vi "Octave Band Frequencies List.vi"(4 "high band selector":i32, 5 "low band selector":i32, 6 "bandwidth":T3(ring)=enum."1/3 octave", 7 "standard":T1) -> (0 "number of bands":i32, 1 "bandedge frequencies [Hz]":T2(array[cluster]) {"midband" format="%.2f"; "f high" format="%.2f"; "f low" format="%.2f"}, 2 "nominal frequencies (string)":string[](array[string]), 3 "nominal frequencies [Hz]":dbl[](array[numeric]) format="%.2f")   [LabVIEW 2017]
doc: "Returns nominal, or preferred, frequencies and bandedge frequencies based on the specified standard (ANSI or IEC), bandwidth, and low and high band selectors.\nThe frequency range is based on the low and high band selectors. A value of 0 corresponds to the reference frequency of the audio-frequency range, 1 kHz. Each successive value corresponds to the next fractional-octave band. Positive values cover the range above 1 kHz, and negative values cover the range below 1 kHz."
uses:
  <vilib>/addons/_NISVFA/_Shared subVIs/Controls/svc_Octave Standard.ctl
  <vilib>/addons/Sound and Vibration/svt_Octave/SoundVib_Octave.lvlib
  <vilib>/addons/Sound and Vibration/svt_Octave/SoundVib_Octave_2014 standard.lvlib
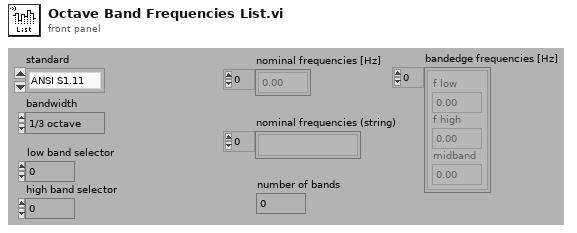
[diagram p1: front panel]
types:
  T1 = typedef "svc_Octave Standard.ctl" = enum16{"ANSI S1.11", "IEC 61260"}
  T2 = cluster{"f low":dbl, "f high":dbl, "midband":dbl}[]
  T3 = enum16{"1 octave", "1/3 octave", "1/6 octave", "1/12 octave", "1/24 octave"}
  T4 = cluster{"f low":dbl, "f high":dbl, "midband frequency [Hz]":dbl}
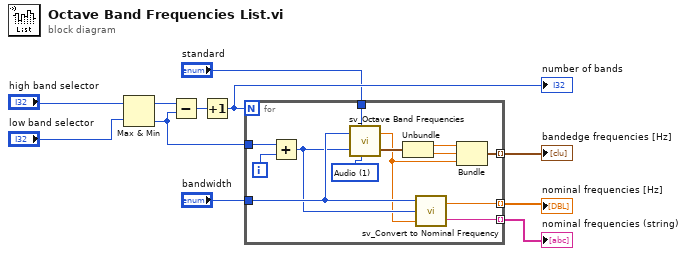
[diagram p0: block diagram]
diagram:
  n1 = Max & Min(x="high band selector", y="low band selector") -> (max(x,y)=w4:i32, min(x,y)=w3:i32)
  n2 = Subtract(x=w4, y=w3) -> (x-y=w11:i32)
  n3 = Increment(x=w11) -> (x+1=w10:i32)
  "number of bands" <- w10
  n4 = for {
    N: w10 -> [_]
    tunnel: w3 -> [w24]
    tunnel: "bandwidth" -> [w16]
    tunnel: [w18] -> w8 mode=indexing
    tunnel: "standard" -> [w17]
    tunnel: [w13] -> w6 mode=indexing
    tunnel: [w12] -> w5 mode=indexing
    i -> [w23]
    w22 = u16 1 items=["Infrasonic", "Audio", "Ultrasonic"] ("Frequency range")
    n5 = Add(x=w24, y=w23) -> (x+y=w15:i32)
    n6 = call <vilib>:"sv_Octave Band Frequencies.vi"("octave band selector"=w15, "reference frequency range"=w22, "bandwidth"=w16, "standard"=w17) -> ("bandedge frequencies [Hz]"=w21:cluster{"f low":dbl, "f high":dbl}, "midband frequency [Hz]"=w14:dbl)  [unwired: 2 out]
    n7 = Unbundle(w21) -> ("f low"=w20:dbl, "f high"=w19:dbl)
    n8 = call <vilib>:"sv_Convert to Nominal Frequency.vi"("bandwidth"=w16, "octave band selector"=w15, "midband frequency [Hz]"=w14) -> ("nominal frequency [Hz]"=w13:dbl, "nominal frequency (string)"=w12:string)  [unwired: 2 in]
    n9 = Bundle("f low"=w20, "f high"=w19, "midband frequency [Hz]"=w14) -> (w18:T4)  [unwired: 1 in]
  }
  "nominal frequencies [Hz]" <- w6
  "bandedge frequencies [Hz]" <- w8
  "nominal frequencies (string)" <- w5
